vi "Safe Trim.vi"(11 "string in":string) -> (3 "result string":string)   [LabVIEW 2020, in "Approval Tests.lvlib"]
uses:
  Approval Tests.lvlib
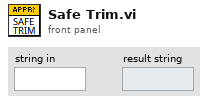
[diagram p1: front panel]
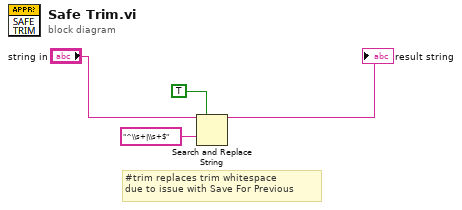
[diagram p0: block diagram]
diagram:
  # "#trim replaces trim whitespace\ndue to issue with Save For Previous"
  n1 = Search and Replace String(replace all?=TRUE ("replace all? (F)"), input string="string in", search string="^\\s+|\\s+$" ("regular expression")) -> (result string=→"result string":string)  [unwired: 5 in, 3 out]
